vi "Read Target.vi"(8 "error in (no error)":errorcluster, 11 "Simple Linked List Task in":refnum<class "Simple Linked List Task.lvclass">) -> (0 "error out":errorcluster, 2 "Target":u32, 3 "Simple Linked List Task out":refnum<class "Simple Linked List Task.lvclass">)   [LabVIEW 2024, in "Simple Linked List Task.lvclass"]
uses:
  Simple Linked List Task.lvclass
  Simple Linked List Task.lvclass/Simple Linked List Task.ctl
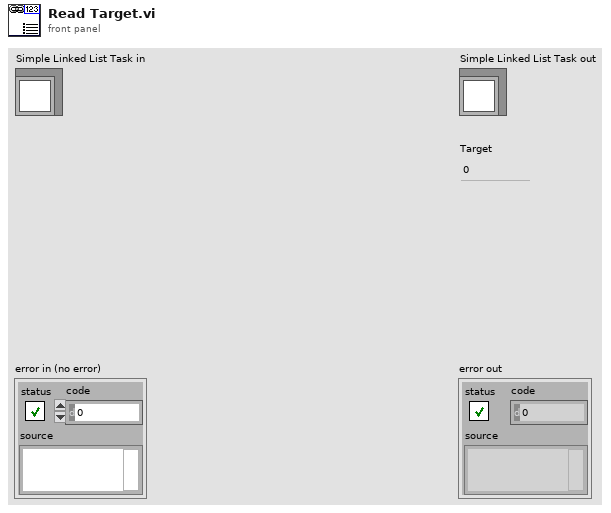
[diagram p1: front panel]
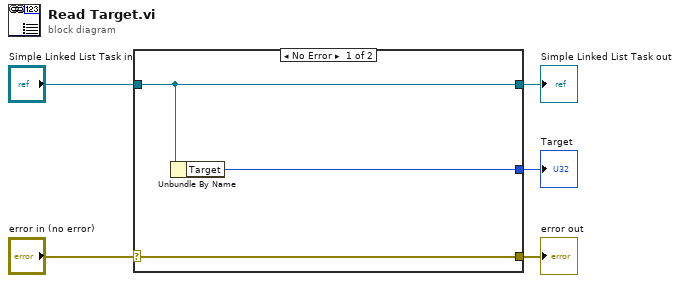
[diagram p0: block diagram]
diagram:
  n1 = case shown="No Error" "error in (no error)" {
    selector: "error in (no error)" -> [w8 w9]
    tunnel: [w8 w9] -> w4
    tunnel: [w7 w10] -> w2
    tunnel: "Simple Linked List Task in" -> [w7 w10]
    tunnel: [w6 _] -> w1
    frame No Error {
      n2 = Unbundle By Name(w7) -> ("Target"=w6:u32)
    }
    frame Error {
    }
  }
  "error out" <- w4
  "Simple Linked List Task out" <- w2
  "Target" <- w1
